vi "Subvi pixel clock generator.vi"(9 "Nmax lines":u16) -> ()   [LabVIEW 2017]
uses:
  <vilib>/Platform/TimedLoop/XDataNode/timing_clust.ctl
  <vilib>/Platform/TimedLoop/XDataNode/nitl_modes.ctl
  <vilib>/Platform/TimedLoop/XDataNode/wakeup.ctl
  <vilib>/rvi/Emulation/niFpgaSctlEmulationGetInTimedLoop.vi
  <vilib>/rvi/Emulation/niFpgaEmulationReportErrorSimple.vi
  <vilib>/rvi/Emulation/niFpgaGetClockAttributes.vi
  <vilib>/rvi/Emulation/niFpgaCriticalErrorInLSC.vi
  <vilib>/rvi/eio/common/nirviEmuTemplateMethod_errors.vi
  GV start acquisition.vi
  <vilib>/rvi/Emulation/niFpgaProcessEmulError.vi
  GV N pixel clock per line.vi
  <vilib>/rvi/Memory/Memory_Emulation/nirvimemoryFastEmulation.vi
  <vilib>/rvi/Memory/Memory_Emulation/nirvimemoryEmulation.vi
  <vilib>/rvi/Emulation/niFpgaEmulationIsFPGAContextNoSignature.vi
  <vilib>/rvi/DataTransferAndStorage/Container/Common/niFpgaContainerGetUniqueNameForEmu.vi
  <vilib>/rvi/errors/nirviReportUnexpectedCaseInternalError (U32).vi
  <vilib>/Platform/TimedLoop/XDataNode/XDataNode.xnode
  <vilib>/eio/EIONode/EIONode.xnode
  <vilib>/rvi/DataTransferAndStorage/Container/XNode/niFpgaContainer.xnode
  <vilib>/Platform/TimedLoop/XDataNode/XDNodeRunTimeDep.lvlib
  GV gated pixel clock change.vi
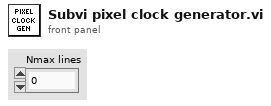
[diagram p1: front panel]
types:
  T1 = typedef "XDNodeRunTimeDep.lvlib/timing_clust.ctl" = cluster{"Expected End [f-1]":u64, "Actual End [f-1]":u64, "Finished Late? [f-1]":bool, "Expected End [i-1]":u64, "Actual End [i-1]":u64, "Finished Late? [i-1]":bool, "Expected Start [i]":u64, "Actual Start [i]":u64, "Expected Start [f]":u64, "Actual Start [f]":u64, "Source Name":string, "Structure Name":string, "Period":i64, "Deadline":i64, "Offset":i64, "Start":i64, "Priority":i32, "Timeout":i32, "Mode":T2, "Wakeup Reason":T3, "Error":errorcluster, "Source Type":string, "Secondary Source Type":string, "Global End Time":u64, "Global Start Time":u64, "Frame Duration":u64, "Iteration Duration":u64, "Assigned CPU":i32, "I/O Scan Engine Mode":u32}
  T2 = typedef "XDNodeRunTimeDep.lvlib/nitl_modes.ctl" = enum32{"No Change", "Process missed periods, maintain original phase", "Discard missed periods, maintain original phase", "Process missed periods, ignore original phase", "Discard missed periods, ignore original phase"}
  T3 = typedef "XDNodeRunTimeDep.lvlib/wakeup.ctl" = enum32{"Normal", "Aborted", "Asynchronous wakeup", "Timing source error", "Timed loop error", "Timeout"}
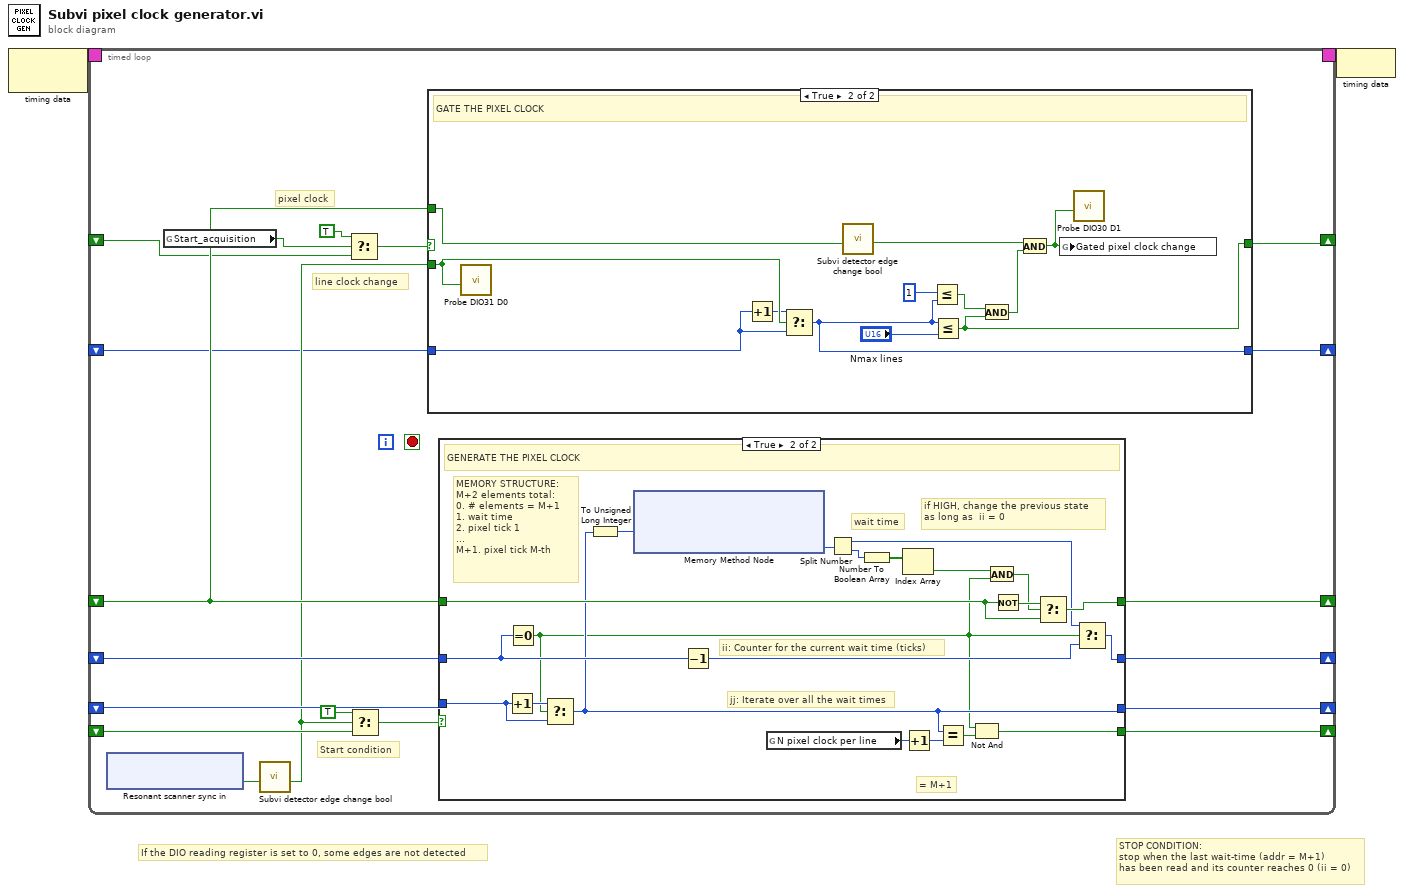
[diagram p0: block diagram]
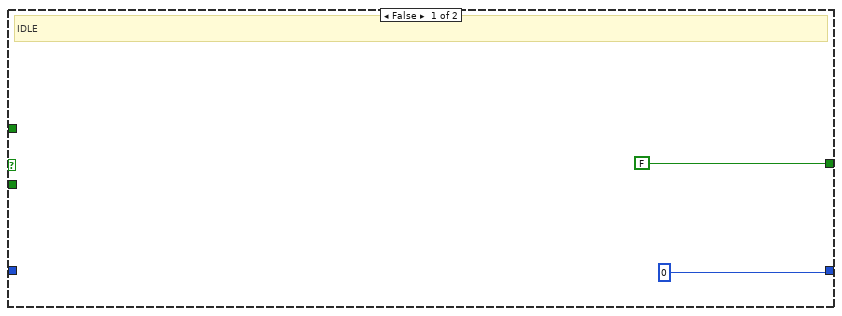
[diagram p2: hidden frame]
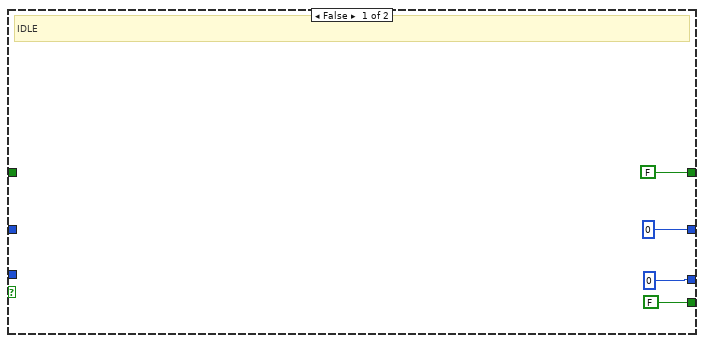
[diagram p3: hidden frame]
diagram:
  # "If the DIO reading register is set to 0, some edges are not detected"
  # "STOP CONDITION:\nstop when the last wait-time (addr = M+1) \nhas been read and its counter reaches 0 (ii = 0)"
  n1 = node-c288() -> (w2:T1)  [unwired: 1 in]
  n2 = timed-loop {
    timing: w2 -> [_]
    timing-out: [_] -> w1
    shift-right: [w19] -> _
    shift-left: _ -> [w20]
    shift-right: [w13] -> _
    shift-left: _ -> [w17]
    shift-right: [w18] -> _
    shift-left: _ -> [w11]
    shift-right: [w15] -> _
    shift-left: _ -> [w16]
    shift-right: [w5] -> _
    shift-left: _ -> [w6]
    shift-right: [w3] -> _
    shift-left: _ -> [w4]
    stop <- _ stop-if-true
    # "line clock change"
    # "pixel clock"
    # "Start condition"
    n3 = xnode "Resonant scanner sync in"() -> ("Connector0/DIO0"=w12:bool)  [unwired: 1 in, 1 out]
    n4 = global read "GV start acquisition.vi" "Start_acquisition"() -> (w9:bool)
    n5 = call "Subvi detector edge change bool.vi"("Input"=w12) -> ("Output"=w10:bool)  [unwired: 8 in]
    n6 = Select(t=TRUE, s=w9, f=w6) -> (s? t:f=w7:bool)
    n7 = Select(t=TRUE, s=w10, f=w17) -> (s? t:f=w14:bool)
    n8 = case shown="True" w7 {
      tunnel: w11 -> [_ w35]
      tunnel: w10 -> [_ w34]
      tunnel: [FALSE w24] -> w5
      tunnel: w4 -> [_ w29]
      tunnel: [u16 0 w28] -> w3
      frame False {
        # "IDLE"
      }
      frame True {
        # "GATE THE PIXEL CLOCK"
        n9 = call "Probe DIO31 D0.vi"("D0"=w34) -> ()  [unwired: 11 in]
        n10 = Increment(x=w29) -> (x+1=w32:u16)
        n11 = Select(t=w32, s=w34, f=w29) -> (s? t:f=w28:u16)
        n12 = call "Subvi detector edge change bool.vi"("Input"=w35) -> ("Output"=w30:bool)  [unwired: 8 in]
        n13 = Less Or Equal?(x=u16 1 ("Min"), y=w28) -> (x <= y?=w26:bool)
        n14 = Less Or Equal?(x=w28, y="Nmax lines") -> (x <= y?=w24:bool)
        n15 = And(x=w26, y=w24) -> (x .and. y?=w25:bool)
        n16 = And(x=w30, y=w25) -> (x .and. y?=w33:bool)
        n17 = global write "GV gated pixel clock change.vi" "Gated pixel clock change"(w33) -> ()
        n18 = call "Probe DIO30 D1.vi"("D1"=w33) -> ()  [unwired: 11 in]
      }
    }
    n19 = case shown="True" w14 {
      tunnel: [FALSE w40] -> w13
      tunnel: w20 -> [_ w52]
      tunnel: [u16 0 w55] -> w19
      tunnel: [FALSE w56] -> w18
      tunnel: w11 -> [_ w53]
      tunnel: w16 -> [_ w51]
      tunnel: [u16 0 w50] -> w15
      frame False {
        # "IDLE"
      }
      frame True {
        # "jj: Iterate over all the wait times"
        # "ii: Counter for the current wait time (ticks)"
        # "MEMORY STRUCTURE:\nM+2 elements total:\n0. # elements = M+1\n1. wait time \n2. pixel tick 1\n...\nM+1. pixel tick M-th"
        # "if HIGH, change the previous state\nas long as  ii = 0"
        # "= M+1"
        # "wait time"
        # "GENERATE THE PIXEL CLOCK"
        n20 = Increment(x=w51) -> (x+1=w60:u16)
        n21 = Equal To 0?(x=w52) -> (x = 0?=w41:bool)
        n22 = Select(t=w60, s=w41, f=w51) -> (s? t:f=w50:u16)
        n23 = To Unsigned Long Integer(number=w50) -> (unsigned 32bit integer=w48:u32)
        n24 = xnode ("Memory Method Node")("Address"=w48) -> ("Data"=w47:u32)  [unwired: 1 in, 1 out]
        n25 = Decrement(x=w52) -> (x-1=w49:u16)
        n26 = global read "GV N pixel clock per line.vi" "N pixel clock per line"() -> (w46:u16)
        n27 = Split Number(x=w47) -> (hi(x)=w54:u16, lo(x)=w58:u16)
        n28 = Number To Boolean Array(number=w58) -> (Boolean array=w59:bool[])
        n29 = Index Array(array=w59) -> (element=w42:bool)  [unwired: 1 in]
        n30 = Increment(x=w46) -> (x+1=w45:u16)
        n31 = Equal?(x=w50, y=w45) -> (x = y?=w44:bool)
        n32 = Not And(1:w44, 2:w41) -> (0:w40:bool)
        n33 = And(x=w42, y=w41) -> (x .and. y?=w43:bool)
        n34 = Not(x=w53) -> (.not. x?=w57:bool)
        n35 = Select(t=w57, s=w43, f=w53) -> (s? t:f=w56:bool)
        n36 = Select(t=w54, s=w41, f=w49) -> (s? t:f=w55:u16)
      }
    }
  }
  n37 = node-c288(w1) -> ()
